vi "UI Backgroud Event.vi"(8 "error in (no error)":errorcluster, 10 "Controls[]":refnum<vi>[](array[refnum]), 11 "Notifier":refnum<notifier>) -> (0 "error out":errorcluster)   [LabVIEW 2015]
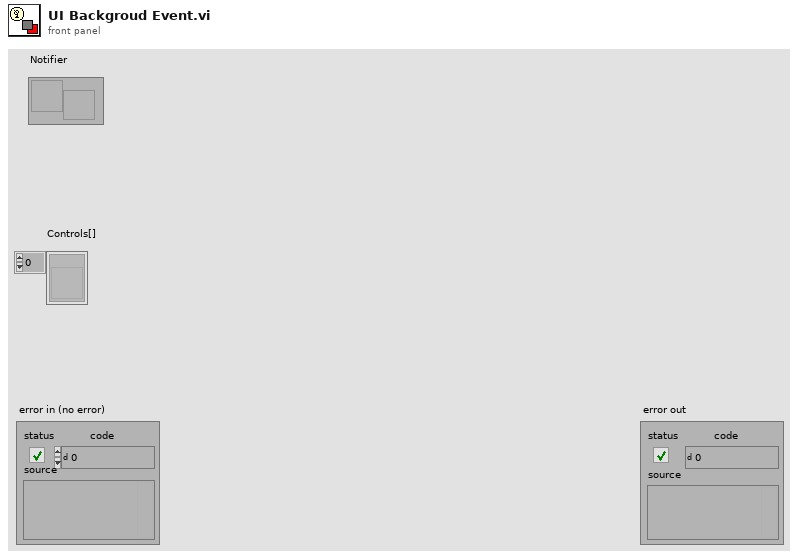
[diagram p1: front panel]
types:
  T1 = cluster{"Event Registration Refnum":refnum<event-registration>, "Ctl Refnum":refnum<vi>}[]
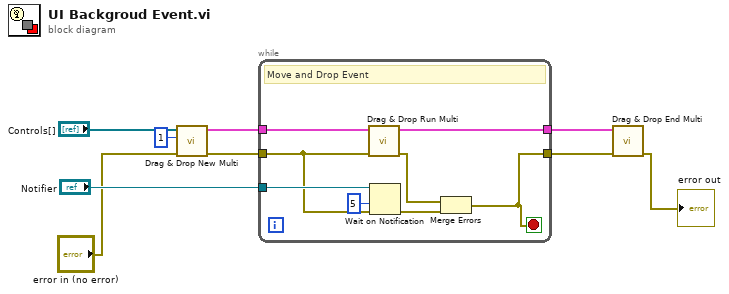
[diagram p0: block diagram]
diagram:
  n1 = call "Drag & Drop New Multi.vi"("References In"="Controls[]", "Index Panel"=1, "error in"="error in (no error)") -> ("References Out"=w8:T1, "error out"=w7:errorcluster)  [unwired: 6 in]
  n2 = while {
    tunnel: w8 -> [w17]
    tunnel: w7 -> [w13]
    tunnel: [w16] -> w6
    tunnel: [w10] -> w5
    tunnel: "Notifier" -> [w15]
    stop <- w10 stop-if-true
    # "Move and Drop Event"
    n3 = call "Drag & Drop Run Multi.vi"("References In"=w17, "error in"=w13) -> ("References Out"=w16:T1, "error out"=w12:errorcluster)  [unwired: 6 in]
    n4 = Wait on Notification(notifier=w15, timeout in ms (-1)=5, error in (no error)=w13) -> (error out=w11:errorcluster)  [unwired: 1 in, 3 out]
    n5 = Merge Errors(w12, w11) -> (w10:errorcluster)
  }
  n6 = call "Drag & Drop End Multi.vi"("errorin"=w5, "References In"=w6) -> ("error out"=→"error out":errorcluster)  [unwired: 9 in]
